vi "Halte_linke_Anschlagssignal_fuer_1sec.vi"(3 "Zeit seit letztem Aufruf":u32, 4 "Banddaten":bool[](array[boolean])=[FALSE, FALSE, FALSE, FALSE, FALSE, FALSE, FALSE, FALSE], 5 "Band-Index":u8) -> (1 "veränderte Banddaten":bool[](array[boolean]))   [LabVIEW 2013]
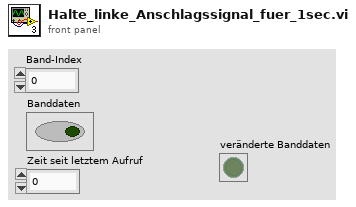
[diagram p1: front panel]
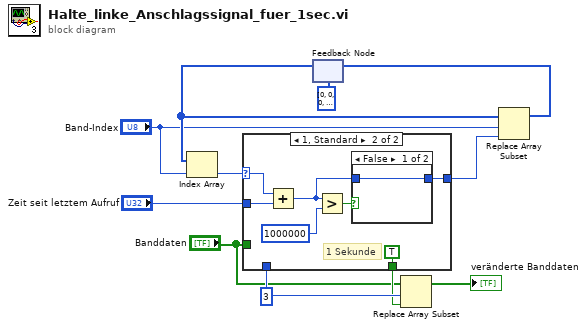
[diagram p0: block diagram]
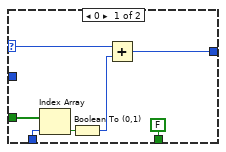
[diagram p2: hidden frame]
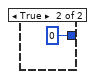
[diagram p3: hidden frame]
diagram:
  w7 = 3 ("Index")
  n1 = feedback #1 ("Rückkopplungsknoten")(u32[] [0, 0, 0, 0, 0, 0, 0, 0, 0, 0]) -> (w10:u32[])
  n2 = Index Array(array=w10, index="Band-Index") -> (element=w4:u32)
  n3 = case shown="1, Standard" w4 {
    selector: w4 -> [w16 w21]
    tunnel: "Banddaten" -> [w18 _]
    tunnel: [w14 w20] -> w5
    tunnel: "Zeit seit letztem Aufruf" -> [_ w25]
    tunnel: w7 -> [w13 _]
    tunnel: [FALSE TRUE] -> w6
    frame 0 {
      n4 = Index Array(array=w18, index=w13) -> (element=w17:bool)
      n5 = Boolean To (0,1)(Boolean=w17) -> (0, 1=w15:i16)
      n6 = Add(x=w16, y=w15) -> (x+y=w14:u32)
    }
    frame 1, Default {
      # "1 Sekunde"
      n7 = Add(x=w21, y=w25) -> (x+y=w19:u32)
      n8 = Greater?(x=w19, y=u32 1000000) -> (0:w22:bool)
      n9 = case shown="False" w22 {
        tunnel: w19 -> [w26 _]
        tunnel: [w26 u32 0 ("Numerisch")] -> w20
        frame False {
        }
        frame True {
        }
      }
    }
  }
  n10 = Replace Array Subset(array="Banddaten", new element=w6, index=w7) -> (→"veränderte Banddaten":bool[])
  n11 = Replace Array Subset(array=w10, new element=w5, index="Band-Index") -> (w9:u32[])
  n12 = feedback-in #1(w9) -> ()
